vi "Look in Map.vi"(9 "default value":refnum<class "IMessagePackObject.lvclass">, 10 "key":refnum<class "IMessagePackObject.lvclass">, 11 "MsgPackMap in":refnum<class "MsgPackMap.lvclass">) -> (1 "value":refnum<class "IMessagePackObject.lvclass">, 2 "key not found?":bool)   [LabVIEW 2020, in "MessagePack.lvlib" / "MsgPackMap.lvclass"]
uses:
  MsgPackMap.lvclass
  MsgPackMap.lvclass/MsgPackMap.ctl
  IMessagePackObject/IMessagePackObject.lvclass
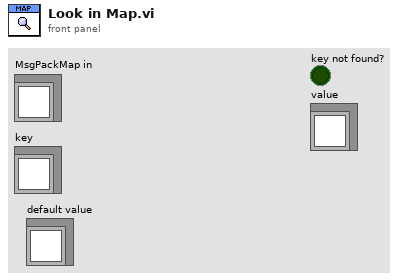
[diagram p1: front panel]
types:
  T1 = map{refnum<class "IMessagePackObject.lvclass">, refnum<class "IMessagePackObject.lvclass">}
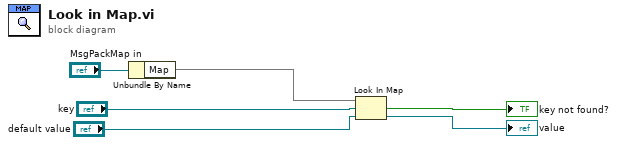
[diagram p0: block diagram]
diagram:
  n1 = Unbundle By Name("MsgPackMap in") -> ("Map"=w3:T1)
  n2 = Look In Map(map=w3, key="key", default value="default value") -> (key not found?=→"key not found?":bool, value=→"value":refnum<class "IMessagePackObject.lvclass">)
